vi "XY-Data to Dictionary.vi"   [LabVIEW 2016, in "LV-Data.lvclass"]
uses:
  LV-Data.lvclass
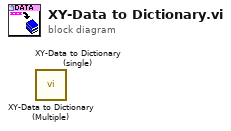
[diagram p0: block diagram]
diagram:
  n1 = call "XY-Data to Dictionary (Multiple).vi"() -> ()  [unwired: 10 in, 2 out]
  n2 = call "XY-Data to Dictionary (single).vi"() -> ()  [unwired: 10 in, 2 out]
